vi "PFD_Top.vi"(8 "Refresh Rate (Hz)":u32=60, 9 "color_palette":T1={"color1"=16777225, "color2"=16777224, "color_line"=16777225}) -> (3 "PFD_Top":picture, 11 "PFD_TopControl":T2={"mav_mode"=1, "ALT"=0.0, "GND ALT"=0.0, "Mission Mode"=21, "Batt Stats"={"Active"=TRUE, "State"=FALSE}, "Sat Stats"={"Active"=TRUE, "State"=FALSE}, "Radio Stats"={"Active"=TRUE, "State"=FALSE}, "Sensor Stats"={"Active"=TRUE, "State"=FALSE}, "SPEED"=0.0, "ASPEED"=0.0, "arm_s"=FALSE})   [LabVIEW 2023]
uses:
  <vilib>/Utility/miscctls.llb/LVBoundsTypeDef.ctl
  PFD_Global.vi
panel:
  in  "stop":bool
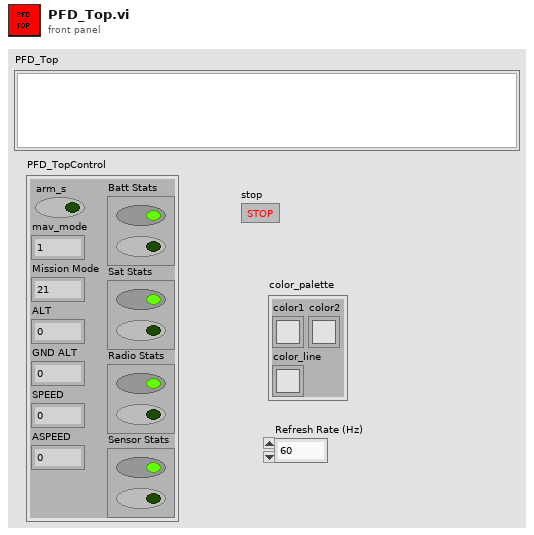
[diagram p1: front panel]
types:
  T1 = cluster{"color1":u32, "color2":u32, "color_line":u32}
  T2 = cluster{"mav_mode":i16, "ALT":dbl, "GND ALT":dbl, "Mission Mode":i16, "Batt Stats":cluster{"Active":bool, "State":bool}, "Sat Stats":cluster{"Active":bool, "State":bool}, "Radio Stats":cluster{"Active":bool, "State":bool}, "Sensor Stats":cluster{"Active":bool, "State":bool}, "SPEED":dbl, "ASPEED":dbl, "arm_s":bool}
  T3 = typedef "LVBoundsTypeDef.ctl" = cluster{"Width":u32, "Height":u32}
  T4 = cluster{"left":i16, "top":i16, "right":i16, "bottom":i16}
  T5 = typedef "imagedata.ctl" = cluster{"image type":i32, "image depth":i32, "image":u8[], "mask":u8[], "colors":u32[], "Rectangle":cluster{"left":i16, "top":i16, "right":i16, "bottom":i16}}
  T6 = cluster{"Font Name:":string, "Size":i16, "Strikeout?":bool, "Italic?":bool, "Underline?":bool, "Outline?":bool, "Shadow?":bool, "Bold?":bool}
  T7 = cluster{"horizontal":enum16{"left", "center", "right"}, "vertical":enum16{"top", "center", "bottom"}}
  T8 = enum16{"User-specified Font", "Application Font", "System Font", "Dialog Font"}
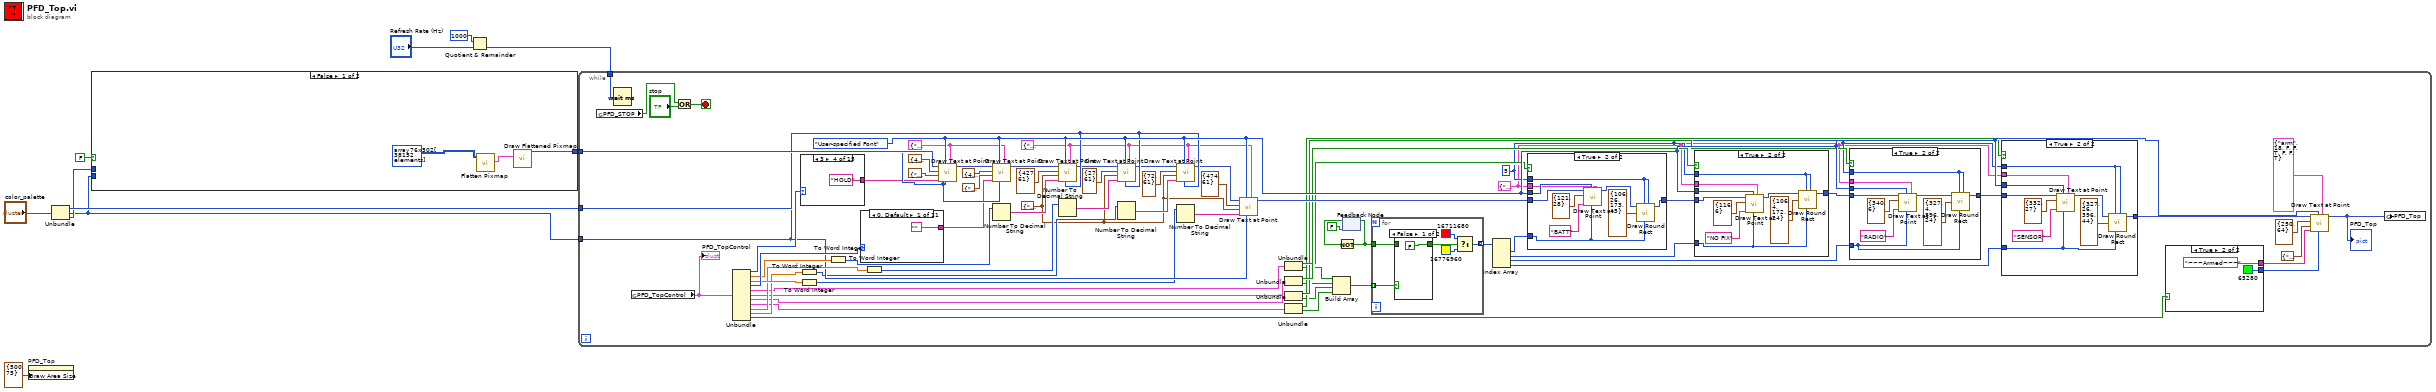
[diagram p0: block diagram]
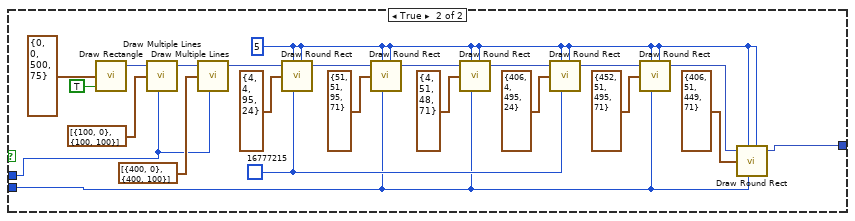
[diagram p2: hidden frame]
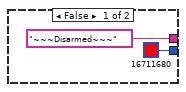
[diagram p3: hidden frame]
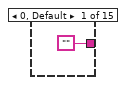
[diagram p9: hidden frame]
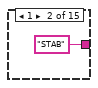
[diagram p10: hidden frame]
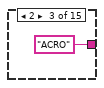
[diagram p11: hidden frame]
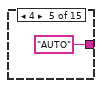
[diagram p12: hidden frame]
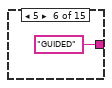
[diagram p13: hidden frame]
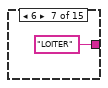
[diagram p14: hidden frame]
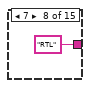
[diagram p15: hidden frame]
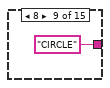
[diagram p16: hidden frame]
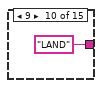
[diagram p17: hidden frame]
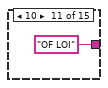
[diagram p18: hidden frame]
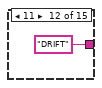
[diagram p19: hidden frame]
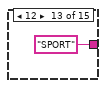
[diagram p20: hidden frame]
diagram:
  n1 = property on="PFD_Top" class="Pict"("Draw Area Size"=T3 {"Width"=500, "Height"=75}) -> ()  [unwired: 2 in, 2 out]
  n2 = Unbundle("color_palette") -> ("color1"=w7:u32, "color2"=w4:u32, "color_line"=w5:u32)
  n3 = case shown="False" FALSE {
    tunnel: [w13 w36] -> w8
    tunnel: w5 -> [_ w15]
    tunnel: w4 -> [_ w14]
    frame False {
      n4 = call <vilib>:"Flatten Pixmap.vi"("24-bit pixmap"=u32[][] array76x502[38152 elements]) -> ("image data"=w11:T5)  [unwired: 10 in]
      n5 = call <vilib>:"Draw Flattened Pixmap.vi"("image data"=w11) -> ("new picture"=w13:picture)  [unwired: 8 in]
    }
    frame True {
      w27 = u32 16777215 ("color(black)")
      w23 = i16 5 ("oval height")
      n6 = call <vilib>:"Draw Rectangle.vi"("rect"=T4 {"left"=0, "top"=0, "right"=500, "bottom"=75}, "fill?(F)"=TRUE) -> ("new picture"=w19:picture)  [unwired: 7 in]
      n7 = call <vilib>:"Draw Multiple Lines.vi"("picture"=w19, "line endpoints"=cluster{"x":i16, "y":i16}[] [{"x"=100, "y"=0}, {"x"=100, "y"=100}], "color(black)"=w15) -> ("new picture"=w18:picture)  [unwired: 6 in]
      n8 = call <vilib>:"Draw Multiple Lines.vi"("picture"=w18, "line endpoints"=cluster{"x":i16, "y":i16}[] [{"x"=400, "y"=0}, {"x"=400, "y"=100}], "color(black)"=w15) -> ("new picture"=w35:picture)  [unwired: 6 in]
      n9 = call <vilib>:"Draw Round Rect.vi"("picture"=w35, "oval width"=w23, "rect"=T4 {"left"=4, "top"=4, "right"=95, "bottom"=24} ("rect 2"), "color(black)"=w27, "oval height"=w23) -> ("new picture"=w33:picture)  [unwired: 4 in]
      n10 = call <vilib>:"Draw Round Rect.vi"("picture"=w33, "oval width"=w23, "rect"=T4 {"left"=51, "top"=51, "right"=95, "bottom"=71} ("rect 4"), "color(black)"=w14, "oval height"=w23) -> ("new picture"=w31:picture)  [unwired: 4 in]
      n11 = call <vilib>:"Draw Round Rect.vi"("picture"=w31, "oval width"=w23, "rect"=T4 {"left"=4, "top"=51, "right"=48, "bottom"=71} ("rect 2"), "color(black)"=w14, "oval height"=w23) -> ("new picture"=w29:picture)  [unwired: 4 in]
      n12 = call <vilib>:"Draw Round Rect.vi"("picture"=w29, "oval width"=w23, "rect"=T4 {"left"=406, "top"=4, "right"=495, "bottom"=24}, "color(black)"=w27, "oval height"=w23) -> ("new picture"=w26:picture)  [unwired: 4 in]
      n13 = call <vilib>:"Draw Round Rect.vi"("picture"=w26, "oval width"=w23, "rect"=T4 {"left"=452, "top"=51, "right"=495, "bottom"=71}, "color(black)"=w14, "oval height"=w23) -> ("new picture"=w24:picture)  [unwired: 4 in]
      n14 = call <vilib>:"Draw Round Rect.vi"("picture"=w24, "oval width"=w23, "rect"=T4 {"left"=406, "top"=51, "right"=449, "bottom"=71} ("rect 3"), "color(black)"=w14, "oval height"=w23) -> ("new picture"=w36:picture)  [unwired: 4 in]
    }
  }
  n15 = Quotient & Remainder(x=u32 1000, y="Refresh Rate (Hz)") -> (floor(x/y)=w1:u32)  [unwired: 1 out]
  n16 = while {
    tunnel: w8 -> [w98]
    tunnel: w7 -> [w93]
    tunnel: w4 -> [w92]
    tunnel: w1 -> [w37]
    stop <- w95 stop-if-true
    w43 = T6 {"Font Name:"="rectangle", "Size"=17, "Strikeout?"=FALSE, "Italic?"=FALSE, "Underline?"=FALSE, "Outline?"=FALSE, "Shadow?"=FALSE, "Bold?"=TRUE} ("[user-specified font] 2")
    w44 = i16 5 ("oval height")
    w89 = T6 {"Font Name:"="rectangle", "Size"=17, "Strikeout?"=FALSE, "Italic?"=FALSE, "Underline?"=FALSE, "Outline?"=FALSE, "Shadow?"=FALSE, "Bold?"=TRUE} ("[user-specified font]")
    w77 = T6 {"Font Name:"="text", "Size"=17, "Strikeout?"=FALSE, "Italic?"=FALSE, "Underline?"=FALSE, "Outline?"=FALSE, "Shadow?"=FALSE, "Bold?"=TRUE} ("[user-specified font]")
    w74 = T7 {"horizontal"=enum."center", "vertical"=enum."center"} ("alignment(left, top)")
    w100 = T8."User-specified Font" ("desired font(Application)")
    n17 = global read "PFD_Global.vi" "PFD_STOP"() -> (w96:bool)
    n18 = Wait (ms)(milliseconds to wait=w37) -> ()  [unwired: 1 out]
    n19 = global read "PFD_Global.vi" "PFD_TopControl"() -> (w91:T2)
    "PFD_TopControl" <- w91
    n20 = Or(x=w96, y="stop") -> (x .or. y?=w95:bool)
    n21 = Unbundle(w91) -> ("mav_mode"=w112:i16, "ALT"=w110:dbl, "GND ALT"=w109:dbl, "Mission Mode"=w111:i16, "Batt Stats"=w103:cluster{"Active":bool, "State":bool}, "Sat Stats"=w104:cluster{"Active":bool, "State":bool}, "Radio Stats"=w105:cluster{"Active":bool, "State":bool}, "Sensor Stats"=w106:cluster{"Active":bool, "State":bool}, "SPEED"=w108:dbl, "ASPEED"=w107:dbl, "arm_s"=w99:bool)
    n22 = To Word Integer(number=w107) -> (16bit integer=w81:i16)
    n23 = To Word Integer(number=w109) -> (16bit integer=w75:i16)
    n24 = case shown="3" w112 {
      tunnel: ["" "STAB" ("text") "ACRO" ("text") "HOLD" ("text") "AUTO" ("text") "GUIDED" ("text") "LOITER" ("text") "RTL" ("text") "CIRCLE" ("text") "LAND" ("text") "OF LOI" ("text") "DRIFT" ("text") "SPORT" ("text") "HYBRID" ("text") "TAOFF" ("text")] -> w70
      frame 0, Default {
      }
      frame 1 {
      }
      frame 2 {
      }
      frame 3 {
      }
      frame 4 {
      }
      frame 5 {
      }
      frame 6 {
      }
      frame 7 {
      }
      frame 8 {
      }
      frame 9 {
      }
      frame 10 {
      }
      frame 11 {
      }
      frame 12 {
      }
      frame 13 {
      }
      frame 22 {
      }
    }
    n25 = To Word Integer(number=w110) -> (16bit integer=w85:i16)
    n26 = case shown="0, Default" w111 {
      tunnel: ["" "NAV" ("text") "LOITER" ("text") "LOITER" ("text") "LOITER" ("text") " RTL" ("text") "LAND" ("text") "TAOFF" ("text") " ROI" ("text") "LAND" ("text") "NAV" ("text")] -> w68
      frame 0, Default {
      }
      frame 16 {
      }
      frame 17 {
      }
      frame 18 {
      }
      frame 19 {
      }
      frame 20 {
      }
      frame 21 {
      }
      frame 22 {
      }
      frame 80 {
      }
      frame 81 {
      }
      frame 82 {
      }
    }
    n27 = To Word Integer(number=w108) -> (16bit integer=w84:i16)
    n28 = call <vilib>:"Draw Text at Point.vi"("[user-specified font]"=w89, "text color(black)"=w93, "desired font(Application)"=w100, "text"=w70, "alignment(left, top)"=T7 {"horizontal"=enum."center", "vertical"=enum."center"}, "origin"=cluster{"x":i16, "y":i16} {"x"=48, "y"=14} ("origin 3"), "picture"=w98) -> ("new picture"=w69:picture)  [unwired: 3 in, 1 out]
    n29 = call <vilib>:"Draw Text at Point.vi"("[user-specified font]"=w89, "text color(black)"=w93, "desired font(Application)"=w100, "text"=w68, "alignment(left, top)"=T7 {"horizontal"=enum."center", "vertical"=enum."center"}, "origin"=cluster{"x":i16, "y":i16} {"x"=448, "y"=14} ("origin 2"), "picture"=w69) -> ("new picture"=w65:picture)  [unwired: 3 in, 1 out]
    n30 = Number To Decimal String(number=w85) -> (decimal integer string=w90:string)  [unwired: 1 in]
    n31 = call <vilib>:"Draw Text at Point.vi"("[user-specified font]"=w77, "text color(black)"=w92, "desired font(Application)"=w100, "text"=w90, "alignment(left, top)"=w74, "origin"=cluster{"x":i16, "y":i16} {"x"=427, "y"=61}, "picture"=w65) -> ("new picture"=w80:picture)  [unwired: 3 in, 1 out]
    n32 = Number To Decimal String(number=w84) -> (decimal integer string=w87:string)  [unwired: 1 in]
    n33 = call <vilib>:"Draw Text at Point.vi"("[user-specified font]"=w77, "text color(black)"=w92, "desired font(Application)"=w100, "text"=w87, "alignment(left, top)"=w74, "origin"=cluster{"x":i16, "y":i16} {"x"=27, "y"=61} ("origin 2"), "picture"=w80) -> ("new picture"=w79:picture)  [unwired: 3 in, 1 out]
    n34 = Number To Decimal String(number=w81) -> (decimal integer string=w82:string)  [unwired: 1 in]
    n35 = call <vilib>:"Draw Text at Point.vi"("[user-specified font]"=w77, "text color(black)"=w92, "desired font(Application)"=w100, "text"=w82, "alignment(left, top)"=w74, "origin"=cluster{"x":i16, "y":i16} {"x"=72, "y"=61} ("origin 3"), "picture"=w79) -> ("new picture"=w78:picture)  [unwired: 3 in, 1 out]
    n36 = Number To Decimal String(number=w75) -> (decimal integer string=w76:string)  [unwired: 1 in]
    n37 = call <vilib>:"Draw Text at Point.vi"("[user-specified font]"=w77, "text color(black)"=w92, "desired font(Application)"=w100, "text"=w76, "alignment(left, top)"=w74, "origin"=cluster{"x":i16, "y":i16} {"x"=474, "y"=61}, "picture"=w78) -> ("new picture"=w102:picture)  [unwired: 3 in, 1 out]
    n38 = Unbundle(w103) -> ("Active"=w63:bool, "State"=w57:bool)
    n39 = Unbundle(w104) -> ("Active"=w64:bool, "State"=w56:bool)
    n40 = Unbundle(w105) -> ("Active"=w60:bool, "State"=w55:bool)
    n41 = Unbundle(w106) -> ("Active"=w58:bool, "State"=w54:bool)
    n42 = Build Array(w57, w56, w55, w54) -> (w53:bool[])
    n43 = feedback #1(FALSE) -> (w48:bool)
    n44 = Not(x=w48) -> (.not. x?=w47:bool)
    n45 = feedback-in #1(w47) -> ()
    n46 = for {
      tunnel: w53 -> [w119] mode=indexing
      tunnel: [w118] -> w46 mode=indexing
      tunnel: w47 -> [w117]
      n47 = case shown="False" w119 {
        tunnel: [FALSE w124] -> w120
        tunnel: w117 -> [_ w124]
        frame False {
        }
        frame True {
        }
      }
      n48 = Select(t=u32 16711680 ("color(black)"), s=w120, f=u32 16776960 ("color(black)")) -> (s? t:f=w118:u32)
    }
    n49 = Index Array(array=w46) -> (element #1=w52:u32, element #2=w51:u32, element #3=w50:u32, element #4=w49:u32)  [unwired: 4 in]
    n50 = case shown="True" w63 {
      tunnel: w102 -> [w147 w149]
      tunnel: w100 -> [_ w155]
      tunnel: [w147 w156] -> w62
      tunnel: w44 -> [_ w151]
      tunnel: w43 -> [_ w150]
      tunnel: w52 -> [_ w148]
      frame False {
      }
      frame True {
        n51 = call <vilib>:"Draw Text at Point.vi"("[user-specified font]"=w150, "text color(black)"=w148, "desired font(Application)"=w155, "text"="BATT", "origin"=cluster{"x":i16, "y":i16} {"x"=121, "y"=28} ("origin 2"), "picture"=w149) -> ("new picture"=w157:picture)  [unwired: 4 in, 1 out]
        n52 = call <vilib>:"Draw Round Rect.vi"("picture"=w157, "oval width"=w151, "rect"=T4 {"left"=106, "top"=26, "right"=173, "bottom"=45}, "color(black)"=w148, "oval height"=w151) -> ("new picture"=w156:picture)  [unwired: 4 in]
      }
    }
    n53 = case shown="True" w64 {
      tunnel: [w158 w167] -> w61
      tunnel: w100 -> [_ w166]
      tunnel: w43 -> [_ w162]
      tunnel: w62 -> [w158 w161]
      tunnel: w44 -> [_ w160]
      tunnel: w51 -> [_ w159]
      frame False {
      }
      frame True {
        n54 = call <vilib>:"Draw Text at Point.vi"("[user-specified font]"=w162, "text color(black)"=w159, "desired font(Application)"=w166, "text"="NO FIX", "origin"=cluster{"x":i16, "y":i16} {"x"=116, "y"=6}, "picture"=w161) -> ("new picture"=w168:picture)  [unwired: 4 in, 1 out]
        n55 = call <vilib>:"Draw Round Rect.vi"("picture"=w168, "oval width"=w160, "rect"=T4 {"left"=106, "top"=4, "right"=172, "bottom"=24} ("rect 2"), "color(black)"=w159, "oval height"=w160) -> ("new picture"=w167:picture)  [unwired: 4 in]
      }
    }
    n56 = case shown="True" w60 {
      tunnel: w61 -> [w136 w139]
      tunnel: [w136 w137] -> w59
      tunnel: w44 -> [_ w146]
      tunnel: w100 -> [_ w145]
      tunnel: w43 -> [_ w141]
      tunnel: w50 -> [_ w140]
      frame False {
      }
      frame True {
        n57 = call <vilib>:"Draw Text at Point.vi"("[user-specified font]"=w141, "text color(black)"=w140, "desired font(Application)"=w145, "text"="RADIO", "origin"=cluster{"x":i16, "y":i16} {"x"=340, "y"=6} ("origin 2"), "picture"=w139) -> ("new picture"=w138:picture)  [unwired: 4 in, 1 out]
        n58 = call <vilib>:"Draw Round Rect.vi"("picture"=w138, "oval width"=w146, "rect"=T4 {"left"=327, "top"=4, "right"=396, "bottom"=24}, "color(black)"=w140, "oval height"=w146) -> ("new picture"=w137:picture)  [unwired: 4 in]
      }
    }
    n59 = case shown="True" w58 {
      tunnel: w59 -> [w125 w128]
      tunnel: [w125 w126] -> w101
      tunnel: w44 -> [_ w135]
      tunnel: w100 -> [_ w129]
      tunnel: w43 -> [_ w131]
      tunnel: w49 -> [_ w130]
      frame False {
      }
      frame True {
        n60 = call <vilib>:"Draw Text at Point.vi"("[user-specified font]"=w131, "text color(black)"=w130, "desired font(Application)"=w129, "text"="SENSOR", "origin"=cluster{"x":i16, "y":i16} {"x"=332, "y"=27} ("origin 3"), "picture"=w128) -> ("new picture"=w127:picture)  [unwired: 4 in, 1 out]
        n61 = call <vilib>:"Draw Round Rect.vi"("picture"=w127, "oval width"=w135, "rect"=T4 {"left"=327, "top"=26, "right"=396, "bottom"=44}, "color(black)"=w130, "oval height"=w135) -> ("new picture"=w126:picture)  [unwired: 4 in]
      }
    }
    n62 = case shown="True" w99 {
      tunnel: ["~~~Disarmed~~~" ("text 2") "~~~Armed~~~" ("text")] -> w40
      tunnel: [u32 16711680 ("text color(black)") u32 65280 ("text color(black)")] -> w39
      frame False {
      }
      frame True {
      }
    }
    n63 = call <vilib>:"Draw Text at Point.vi"("[user-specified font]"=T6 {"Font Name:"="arm", "Size"=18, "Strikeout?"=FALSE, "Italic?"=FALSE, "Underline?"=TRUE, "Outline?"=FALSE, "Shadow?"=FALSE, "Bold?"=TRUE}, "text color(black)"=w39, "desired font(Application)"=w100, "text"=w40, "alignment(left, top)"=T7 {"horizontal"=enum."center", "vertical"=enum."center"}, "origin"=cluster{"x":i16, "y":i16} {"x"=250, "y"=64}, "picture"=w101) -> ("new picture"=w94:picture)  [unwired: 3 in, 1 out]
    "PFD_Top" <- w94
    n64 = global write "PFD_Global.vi" "PFD_Top"(w94) -> ()
  }
